vi "Close Module.vi"(8 "error in":errorcluster, 9 "Wait for stop?":bool, 11 "Module Admin in":refnum<class "Delacor_lib_QMH_Cloneable Module Admin.lvclass">) -> (0 "error out":errorcluster, 1 "External Launch":bool, 3 "Module Admin out":refnum<class "Delacor_lib_QMH_Cloneable Module Admin.lvclass">)   [LabVIEW 2024, in "cameraV1.lvlib"]
doc: "Destroy the Broadcast Events and Request Events (if this was the first instance). Reset flags stored in Module Admin class.\n_____\nBased on DQMH Dev Tools: Project Template 7.1.0.1503."
uses:
  cameraV1.lvlib
  <vilib>/Delacor/Delacor QMH/Libraries/Cloneable Module Admin_class/Delacor_lib_QMH_Cloneable Module Admin.lvclass
  Stop Argument--cluster.ctl
  <vilib>/Delacor/Delacor QMH/Libraries/Cloneable Module Admin_class/Delacor_lib_QMH_Cloneable Module Admin.lvclass/Delacor_lib_QMH_Cloneable Module Admin.ctl
  <vilib>/Delacor/Delacor QMH/Libraries/Module Admin_class/Delacor_lib_QMH_Module Admin.lvclass/Delacor_lib_QMH_Module Admin.ctl
  <vilib>/Delacor/Delacor QMH/Libraries/Cloneable Module Admin_class/Delacor_lib_QMH_Get First.vi
  <vilib>/Delacor/Delacor QMH/Libraries/Cloneable Module Admin_class/Delacor_lib_QMH_Get Module ID.vi
  <vilib>/Delacor/Delacor QMH/Libraries/Module Admin_class/Delacor_lib_QMH_Get External Launch.vi
  <vilib>/Delacor/Delacor QMH/Libraries/Cloneable Module Admin_class/Delacor_lib_QMH_Get Close Master Reference.vi
  Clone Registration/Clone Registration.lvlib
  VI Reference Management/VI Reference Management.lvlib
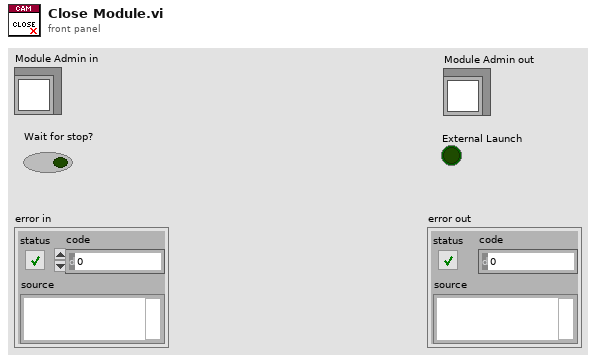
[diagram p1: front panel]
types:
  T1 = typedef "cameraV1.lvlib/Stop Argument--cluster.ctl" = cluster{"Module ID":i32, "Origin":string, "Exit via Stop Module Req?":bool, "Wait for Module to stop?":bool}
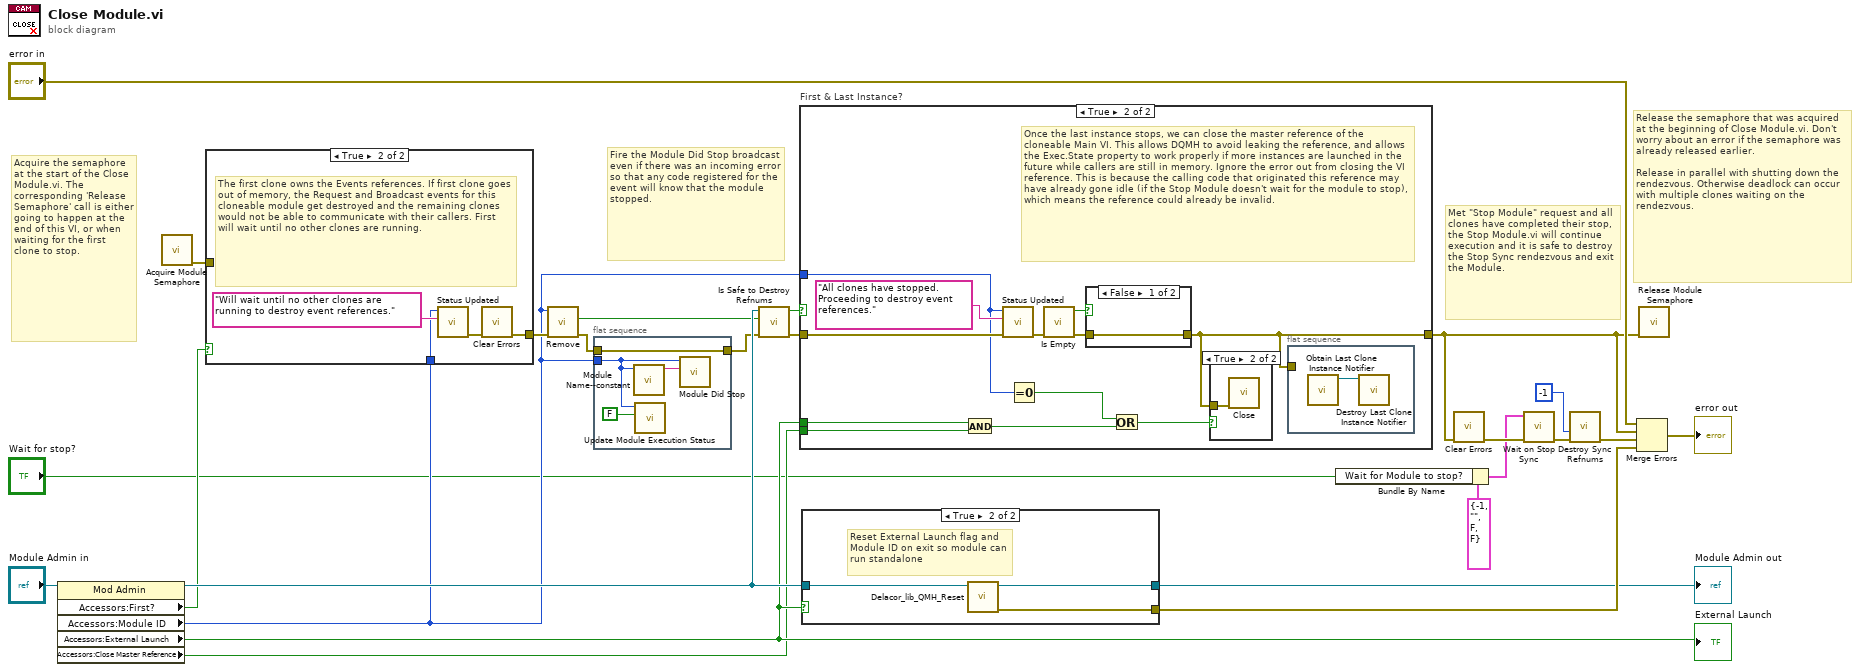
[diagram p0: block diagram]
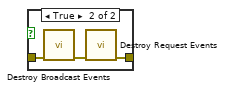
[diagram p5: hidden frame]
diagram:
  # "Release the semaphore that was acquired at the beginning of Close Module.vi. Don't worry about an error if the semaphore was already released earlier.\n\nRelease in parallel with shutting down the rendezvous. Otherwise deadlock can occur with multiple clones waiting on the rendezvous."
  # "Acquire the semaphore at the start of the Close Module.vi. The corresponding 'Release Semaphore' call is either going to happen at the end of this VI, or when waiting for the first clone to stop."
  # "Fire the Module Did Stop broadcast even if there was an incoming error so that any code registered for the event will know that the module stopped."
  # "Met \"Stop Module\" request and all clones have completed their stop, the Stop Module.vi will continue execution and it is safe to destroy the Stop Sync rendezvous and exit the Module."
  n1 = property class="Mod Admin"(reference="Module Admin in") -> (reference out=w23:refnum<class "Delacor_lib_QMH_Cloneable Module Admin.lvclass">, "Accessors:First?"=w14:bool, "Accessors:Module ID"=w8:i32, "Accessors:External Launch"=w12:bool, "Accessors:Close Master Reference"=w7:bool)  [unwired: 1 in, 1 out]
  "External Launch" <- w12
  n2 = call "Acquire Module Semaphore.vi"() -> ("error out"=w6:errorcluster)  [unwired: 11 in]
  n3 = case shown="True" w14 {
    tunnel: w8 -> [_ w28]
    tunnel: [_ w26] -> w25
    tunnel: w6 -> [_ _]
    frame False {
    }
    frame True {
      # "The first clone owns the Events references. If first clone goes out of memory, the Request and Broadcast events for this cloneable module get destroyed and the remaining clones would not be able to communicate with their callers. First will wait until no other clones are running."
      n4 = call "Status Updated.vi"("Status"="Will wait until no other clones are running to destroy event references." ("format string"), "Module ID"=w28) -> ("error out"=w27:errorcluster)  [unwired: 9 in]
      n5 = call <vilib>:"Clear Errors.vi"("error in (no error)"=w27) -> ("error out"=w26:errorcluster)  [unwired: 5 in, 1 out]
    }
  }
  n6 = call "Remove.vi"("error in"=w25, "Module ID"=w8) -> ("error out"=w10:errorcluster, "empty"=w11:bool)  [unwired: 8 in]
  n7 = flat-sequence {
    tunnel: w10 -> [w33]
    tunnel: [w33] -> w9
    tunnel: w8 -> [w31]
    frame #0 {
      n8 = call "Module Name--constant.vi"("Module ID"=w31) -> ("Module Name"=w32:string)  [unwired: 10 in]
      n9 = call "Update Module Execution Status.vi"("Running?"=FALSE, "Module ID"=w31) -> ()  [unwired: 9 in, 1 out]
      n10 = call "Module Did Stop.vi"("Origin"=w32, "Module ID"=w31) -> ()  [unwired: 9 in, 1 out]
    }
  }
  n11 = call "Is Safe to Destroy Refnums.vi"("error in"=w9, "empty"=w11, "Module Admin"=w23) -> ("error out"=w20:errorcluster, "Destroy Broadcast & Request Event Refs?"=w21:bool)  [unwired: 7 in]
  n12 = case "First & Last Instance?" shown="True" w21 {
    tunnel: w20 -> [w34 w46]
    tunnel: [w34 w38] -> w4
    tunnel: w8 -> [_ w40]
    tunnel: w12 -> [_ w44]
    tunnel: w7 -> [_ w42]
    frame False {
    }
    frame True {
      # "Once the last instance stops, we can close the master reference of the cloneable Main VI. This allows DQMH to avoid leaking the reference, and allows the Exec.State property to work properly if more instances are launched in the future while callers are still in memory. Ignore the error out from closing the VI reference. This is because the calling code that originated this reference may have already gone idle (if the Stop Module doesn't wait for the module to stop), which means the reference could already be invalid."
      n13 = And(x=w44, y=w42) -> (x .and. y?=w43:bool)
      n14 = call "Status Updated.vi"("error in"=w46, "Status"="All clones have stopped. Proceeding to destroy event references.", "Module ID"=w40) -> ("error out"=w37:errorcluster)  [unwired: 8 in]
      n15 = Equal To 0?(x=w40) -> (x = 0?=w39:bool)
      n16 = call "Is Empty.vi"("error in"=w37) -> ("error out"=w36:errorcluster, "Empty?"=w35:bool)  [unwired: 9 in]
      n17 = case shown="False" w35 {
        tunnel: [w47 w49] -> w38
        tunnel: w36 -> [w47 w48]
        frame False {
        }
        frame True {
          n18 = call "Destroy Broadcast Events.vi"("error in"=w48) -> ("error out"=w50:errorcluster)  [unwired: 10 in]
          n19 = call "Destroy Request Events.vi"("error in"=w50) -> ("error out"=w49:errorcluster)  [unwired: 10 in]
        }
      }
      n20 = Or(x=w39, y=w43) -> (x .or. y?=w41:bool)
      n21 = case shown="True" w41 {
        tunnel: w38 -> [_ w52]
        frame False {
        }
        frame True {
          n22 = call "Close.vi"("error in"=w52) -> ()  [unwired: 10 in, 1 out]
        }
      }
      n23 = flat-sequence {
        tunnel: w38 -> [_]
        frame #0 {
          n24 = call "Obtain Last Clone Instance Notifier.vi"() -> ("Last Instance Notifier"=w51:refnum<notifier>)  [unwired: 10 in, 1 out]
          n25 = call "Destroy Last Clone Instance Notifier.vi"("Last Instance Notifier"=w51) -> ()  [unwired: 11 in]
        }
      }
    }
  }
  n26 = case shown="True" w12 {
    tunnel: w23 -> [w53 w56]
    tunnel: [w53 w55] -> w19
    tunnel: [_ w54] -> w24
    frame False {
    }
    frame True {
      # "Reset External Launch flag and Module ID on exit so module can run standalone"
      n27 = call-dynamic "Delacor_lib_QMH_Reset.vi"("Mod Admin in"=w56) -> ("error out"=w54:errorcluster, "Mod Admin out"=w55:refnum<class "Delacor_lib_QMH_Cloneable Module Admin.lvclass">)  [unwired: 9 in]
    }
  }
  "Module Admin out" <- w19
  n28 = Bundle By Name(cluster=T1 {"Module ID"=-1, "Origin"="", "Exit via Stop Module Req?"=FALSE, "Wait for Module to stop?"=FALSE} ("Stop Argument"), "Wait for Module to stop?"="Wait for stop?") -> (w2:T1)
  n29 = call <vilib>:"Clear Errors.vi"("error in (no error)"=w4) -> ("error out"=w15:errorcluster)  [unwired: 5 in, 1 out]
  n30 = call "Wait on Stop Sync.vi"("error in"=w15, "Stop Argument"=w2) -> ("error out"=w18:errorcluster)  [unwired: 9 in]
  n31 = call "Destroy Sync Refnums.vi"("error in"=w18, "Module ID"=-1) -> ("error out"=w17:errorcluster)  [unwired: 9 in]
  n32 = Merge Errors("error in", w4, w17, w24) -> (→"error out":errorcluster)
  n33 = call "Release Module Semaphore.vi"("error in"=w4) -> ()  [unwired: 10 in, 1 out]
